vi "Remove next Events.vi"(0 "Note Events in":T1[](array[typedef]), 3 "Event Index":i32) -> (7 "Note Events w/ subset deleted":T1[](array[typedef]), 8 "Note Event Removed":u32, 9 "Note Removed":u32, 10 "Volume Removed":u32)   [LabVIEW 2016]
uses:
  Notes.ctl
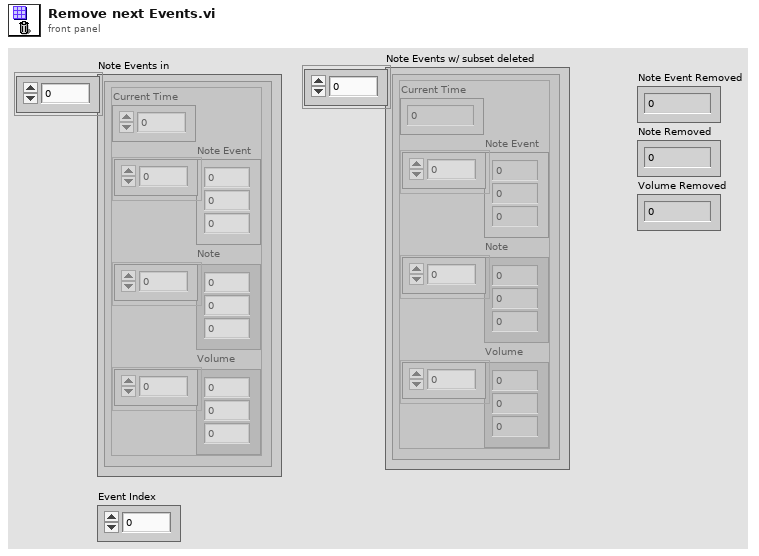
[diagram p1: front panel]
types:
  T1 = typedef "Notes.ctl" = cluster{"Current Time":u32, "Note Event":u32[], "Note":u32[], "Volume":u32[]}
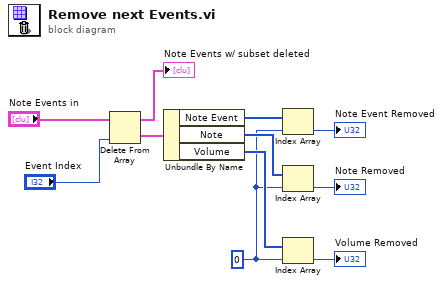
[diagram p0: block diagram]
diagram:
  w4 = 0 ("index")
  n1 = Delete From Array(array="Note Events in", index="Event Index") -> (deleted portion=w9:T1, array with subset deleted=→"Note Events w/ subset deleted":T1[])  [unwired: 1 in]
  n2 = Unbundle By Name(w9) -> ("Note Event"=w7:u32[], "Note"=w6:u32[], "Volume"=w5:u32[])
  n3 = Index Array(array=w7, index=w4) -> (element=→"Note Event Removed":u32)
  n4 = Index Array(array=w6, index=w4) -> (element=→"Note Removed":u32)
  n5 = Index Array(array=w5, index=w4) -> (element=→"Volume Removed":u32)
